vi "Digital_Out_Cmd_v1.vi"(8 "error in (no error)":errorcluster, 10 "DO Command":bool[](array[boolean]), 11 "ControlBoard VISA":refnum<visa-resource-name>="ControlBoard") -> (0 "error out":errorcluster, 3 "ControlBoard VISA Out":refnum<visa-resource-name>)   [LabVIEW 2019]
uses:
  <vilib>/Instr/_visa.llb/VISA Flush IO Buffer Mask.ctl
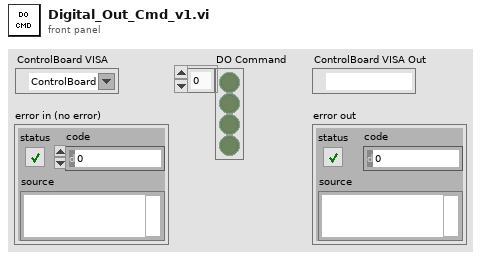
[diagram p1: front panel]
types:
  T1 = typedef "VISA Flush IO Buffer Mask.ctl" = u16
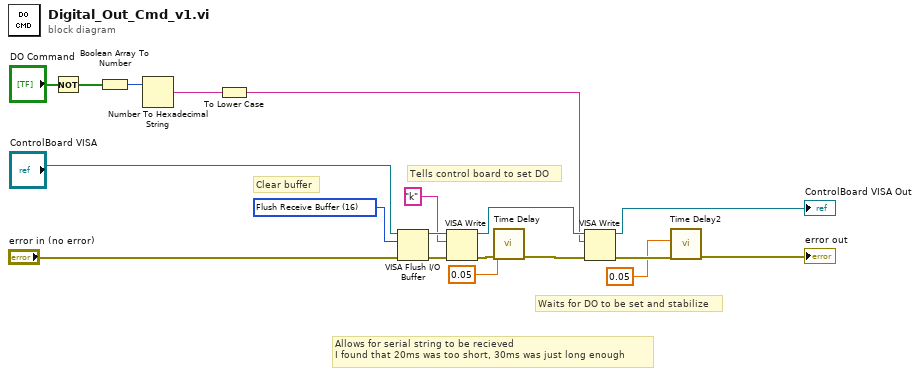
[diagram p0: block diagram]
diagram:
  w15 = T1 16 items=["Flush Receive Buffer"=16, "Write Transmit Buffer to Device"=32, "Flush Receive Buffer (No I/O)"=64, "Flush Transmit Buffer"=128] ("Mask")
  # "Waits for DO to be set and stabilize"
  # "Clear buffer"
  # "Allows for serial string to be recieved\nI found that 20ms was too short, 30ms was just long enough"
  # "Tells control board to set DO"
  n1 = Not(x="DO Command") -> (.not. x?=w6:bool[])
  n2 = Boolean Array To Number(Boolean array=w6) -> (number=w13:u32)
  n3 = Number To Hexadecimal String(2:w13) -> (0:w10:string)  [unwired: 1 in]
  n4 = To Lower Case(string=w10) -> (all lower case string=w7:string)
  n5 = VISA Flush I/O Buffer(VISA resource name="ControlBoard VISA", mask (16)=w15, error in (no error)="error in (no error)") -> (VISA resource name out=w17:refnum<visa-resource-name>, error out=w18:errorcluster)
  n6 = VISA Write(VISA resource name=w17, write buffer="k", error in (no error)=w18) -> (VISA resource name out=w8:refnum<visa-resource-name>, error out=w16:errorcluster)  [unwired: 1 out]
  n7 = call "Time Delay"("error in (no error)"=w16, "Delay Time (s)"=0.05) -> ("error out"=w9:errorcluster)  [unwired: 9 in]
  n8 = VISA Write(VISA resource name=w8, write buffer=w7, error in (no error)=w9) -> (VISA resource name out=→"ControlBoard VISA Out":refnum<visa-resource-name>, error out=w5:errorcluster)  [unwired: 1 out]
  n9 = call "Time Delay2"("error in (no error)"=w5, "Delay Time (s)"=0.05) -> ("error out"=→"error out":errorcluster)  [unwired: 9 in]
